vi "ImageArray2File (SubVI).vi"(5 "Array":dbl[][](array[numeric]), 7 "Save CSV Files Path":path, 8 "error in (no error)":errorcluster, 9 "Image file name ext":string, 10 "Image File Name":string, 11 "Content_ str":string) -> (0 "error out":errorcluster)   [LabVIEW 2016]
uses:
  <vilib>/Utility/file.llb/Write Delimited Spreadsheet (DBL).vi
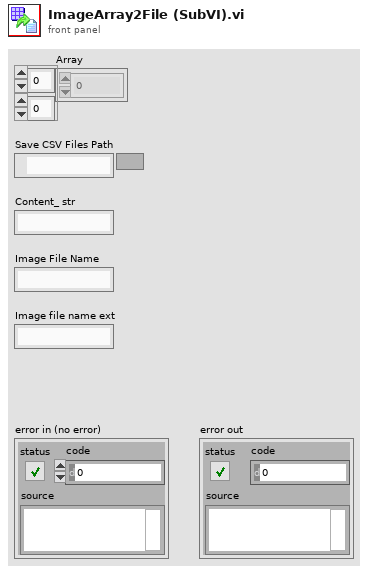
[diagram p1: front panel]
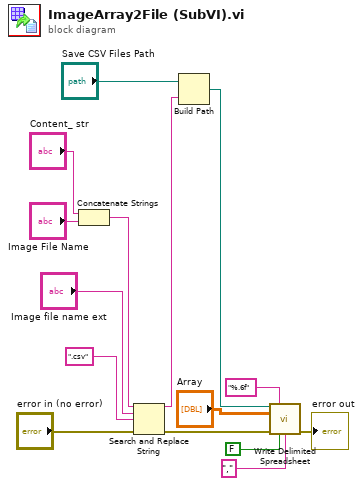
[diagram p0: block diagram]
diagram:
  n1 = Concatenate Strings("Content_ str", "Image File Name") -> (w4:string)
  n2 = Search and Replace String(input string=w4, search string="Image file name ext", replace string=".csv" ("New ext for CSV"), error in="error in (no error)") -> (result string=w5:string, error out=w1:errorcluster)  [unwired: 4 in, 2 out]
  n3 = Build Path(base path="Save CSV Files Path", name or relative path=w5) -> (appended path=w13:path)
  n4 = call-poly <vilib>:"Write Delimited Spreadsheet.vi"("file path (dialog if empty)"=w13, "format (%.3f)"="%.6f", "2D data"="Array", "error in (no error)"=w1, "transpose? (no:F)"=FALSE, "delimiter (\\t)"="," ("delimiter (\\t)")) -> ("error out"=→"error out":errorcluster)  [unwired: 8 in, 1 out]
